vi "PI Convert 1.3 to 1.4.vi"(0 "Prompted Inputs 1.3 Test Parameters":T2={"Tag"="", "Use Instrument"=FALSE, "Quick Mode"=FALSE, "Blank Screen"=FALSE, "Limits"=[], "Datasheets"={"Datasheets to Generate"=[], "Print Datasheets"=TRUE}, "Prompted Items"=[]}) -> (1 "QuickMode":i8, 2 "Prompted Inputs 1.4 Test Parameters":T1)   [LabVIEW 2011]
uses:
  TypeDefs/PI Test Parameters v1.3.ctl
  TypeDefs/PI Test Parameters v1.4.ctl
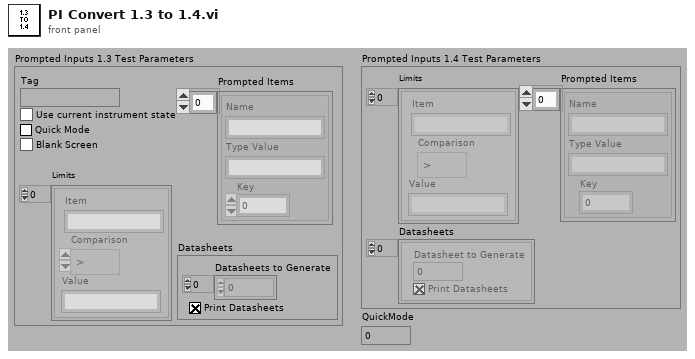
[diagram p1: front panel]
types:
  T1 = typedef "PI Test Parameters v1.4.ctl" = cluster{"Limits":cluster{"Item":string, "Comparison":enum16{">", ">=", "<", "<=", "<>", "="}, "Value":string}[], "Datasheets":cluster{"Datasheet to Generate":i32, "Print Datasheets":bool}[], "Prompted Items":cluster{"Name":string, "Type Value":string, "Key":i32}[]}
  T2 = typedef "PI Test Parameters v1.3.ctl" = cluster{"Tag":string, "Use Instrument":bool, "Quick Mode":bool, "Blank Screen":bool, "Limits":cluster{"Item":string, "Comparison":enum16{">", ">=", "<", "<=", "<>", "="}, "Value":string}[], "Datasheets":cluster{"Datasheets to Generate":i32[], "Print Datasheets":bool}, "Prompted Items":cluster{"Name":string, "Type Value":string, "Key":i32}[]}
  T3 = cluster{"Item":string, "Comparison":enum16{">", ">=", "<", "<=", "<>", "="}, "Value":string}[]
  T4 = cluster{"Name":string, "Type Value":string, "Key":i32}[]
  T5 = cluster{"Datasheet to Generate":i32, "Print Datasheets":bool}[]
  T6 = cluster{"Datasheet to Generate":i32, "Print Datasheets":bool}
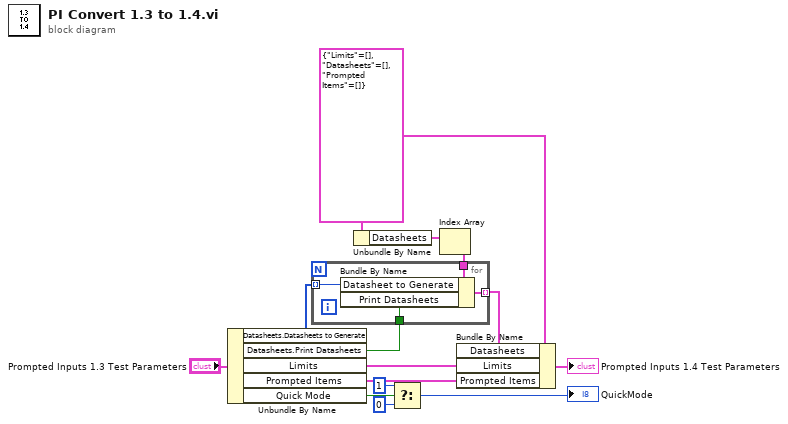
[diagram p0: block diagram]
diagram:
  w7 = T1 {"Limits"=[], "Datasheets"=[], "Prompted Items"=[]} ("Prompted Inputs Test Parameters")
  n1 = Unbundle By Name("Prompted Inputs 1.3 Test Parameters") -> ("Datasheets.Datasheets to Generate"=w11:i32[], "Datasheets.Print Datasheets"=w10:bool, "Limits"=w9:T3, "Prompted Items"=w5:T4, "Quick Mode"=w1:bool)
  n2 = Unbundle By Name(w7) -> ("Datasheets"=w14:T5)
  n3 = Select(t=i8 1 ("QuickMode"), s=w1, f=i8 0 ("QuickMode")) -> (s? t:f=→"QuickMode":i8)
  n4 = Index Array(array=w14) -> (element=w13:T6)  [unwired: 1 in]
  n5 = for {
    tunnel: w13 -> [w18]
    tunnel: [w17] -> w8 mode=indexing
    tunnel: w11 -> [w16] mode=indexing
    tunnel: w10 -> [w15]
    n6 = Bundle By Name(cluster=w18, "Datasheet to Generate"=w16, "Print Datasheets"=w15) -> (w17:T6)
  }
  n7 = Bundle By Name(cluster=w7, "Datasheets"=w8, "Limits"=w9, "Prompted Items"=w5) -> (→"Prompted Inputs 1.4 Test Parameters":T1)
